vi "calc FFT.vi"(8 "dt":dbl=1e-06 format="%#_13g", 9 "Unit":T1, 10 "Window":T2=1 items=["Rectangle"=0, "Hanning"=1, "Hamming"=2, "Blackman-Harris"=3, "Exact Blackman"=4, "Blackman"=5, "Flat Top"=6, "4 Term B-Harris "=7, "7 Term B-Harris"=8, "Low Sidelobe"=9, "Blackman Nuttall"=11, "Triangle"=30, "Bartlett-Hanning"=31, "Bohman"=32, "Parzen"=33, "Welch"=34, "Kaiser"=60, "Dolph-Chebyshev"=61, "Gaussian"=62], 11 "data":dbl[][](array[numeric])) -> (3 "Power Spectrum / PSD":cluster{"f0":dbl, "df":dbl, "magnitude":dbl[]}[](array[cluster]) {"magnitude" format="%.2p"; "f0" format="%.2p"; "df" format="%.2p"})   [LabVIEW 2013]
uses:
  <vilib>/Analysis/4window.llb/windowTd.ctl
  controls/power_spectrum_unit.ctl
  <vilib>/measure/maspectr.llb/Power Spectrum and PSD Export Mode.ctl
  <vilib>/measure/maspectr.llb/FFT Power Spectrum and PSD for N Chan (CDB).vi
  <vilib>/measure/NI_MAPro.lvlib
  <vilib>/Analysis/NI_AALPro.lvlib
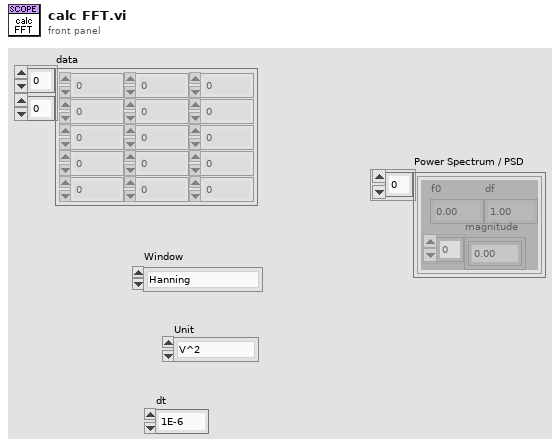
[diagram p1: front panel]
types:
  T1 = typedef "power_spectrum_unit.ctl" = enum16{"V^2", "V", "dBV"}
  T2 = typedef "NI_AALPro.lvlib/windowTd.ctl" = u32
  T3 = typedef "NI_MAPro.lvlib/Power Spectrum and PSD Export Mode.ctl" = u16
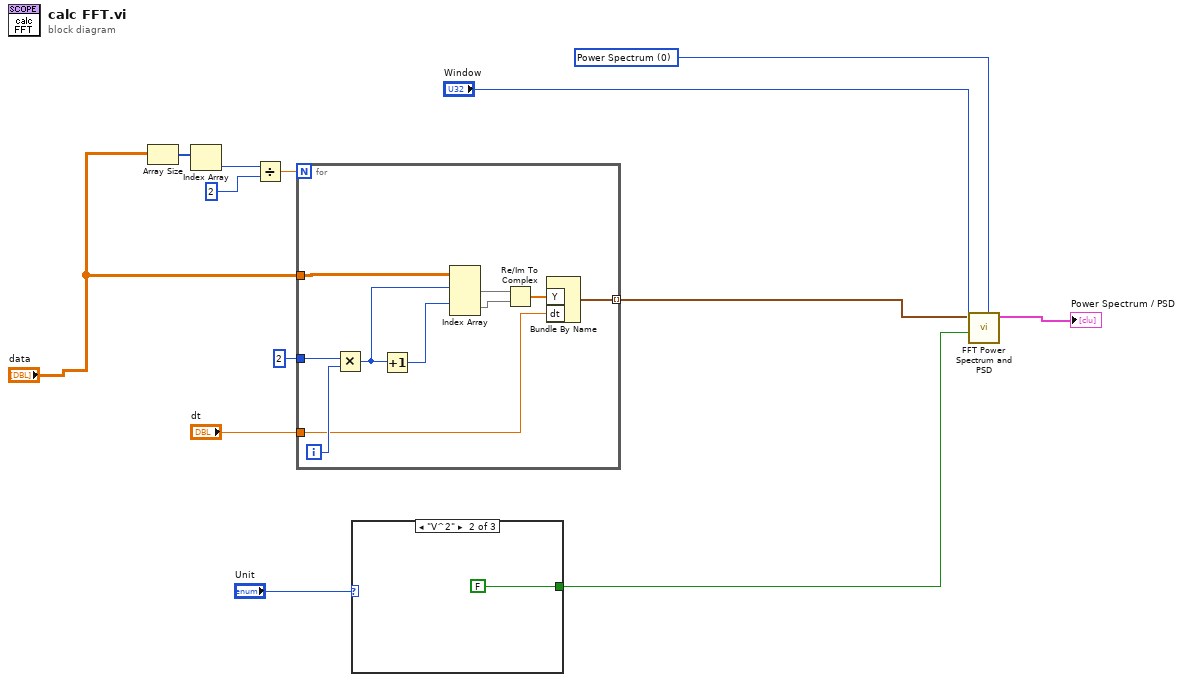
[diagram p0: block diagram]
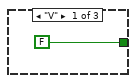
[diagram p2: hidden frame]
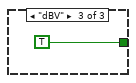
[diagram p3: hidden frame]
diagram:
  w9 = T3 0 items=["Power Spectrum", "Power Spectral Density"] ("export mode")
  n1 = Array Size(array="data") -> (size(s)=w8:i32[])
  n2 = Index Array(array=w8) -> (element=w7:i32)  [unwired: 1 in]
  n3 = Divide(x=w7, y=2) -> (x/y=w4:dbl)
  n4 = for {
    N: w4 -> [_]
    tunnel: "data" -> [w23]
    tunnel: 2 ("y") -> [w22]
    tunnel: [w16] -> w1 mode=indexing
    tunnel: "dt" -> [w14]
    i -> [w15]
    n5 = Multiply(x=w22, y=w15) -> (x*y=w21:i32)
    n6 = Increment(x=w21) -> (x+1=w18:i32)
    n7 = Index Array(array=w23, index (row) #1=w21, index (row) #2=w18) -> (element #1=w19:dbl[], element #2=w17:dbl[])  [unwired: 2 in]
    n8 = Re/Im To Complex(1:w17, 2:w19) -> (0:w20:cdb[])
    n9 = Bundle By Name("Y"=w20, "dt"=w14) -> (w16:waveform(cdb))  [unwired: 1 in]
  }
  n10 = case shown="\"V^2\"" "Unit" {
    tunnel: [FALSE ("dB On (F)") FALSE ("dB On (F)") TRUE ("dB On (F)")] -> w11
    frame "V" {
    }
    frame "V^2" {
    }
    frame "dBV" {
    }
  }
  n11 = call-poly <vilib>:"FFT Power Spectrum and PSD.vi"("export mode"=w9, "dB On (F)"=w11, "window"="Window", "time signals"=w1) -> ("Power Spectrum / PSD"=→"Power Spectrum / PSD":cluster{"f0":dbl, "df":dbl, "magnitude":dbl[]}[])  [unwired: 4 in, 3 out]
